vi "test_SomeSessionsRegistered_CallCreateSessions_InitializeCalledWithProperBehavior.vi"(8 "error in":errorcluster) -> (0 "error out":errorcluster, 2 "result":string, 3 "pass":bool)   [LabVIEW 2020, in "MeasurementServerTests.lvlib"]
uses:
  MeasurementServerTests.lvlib
  da6ffb6f-c1c9-4957-84dd-e9228483c454.vi
  ffc64c76-1568-41a3-8328-b9126ac9a28d.vi
  Helpers/Fake Instrument/Fake Instrument.lvclass
  \\tsclient\C/dev/measurementlink-labview/Source/Runtime/MeasurementLink Instrument/IInstrument/IInstrument.lvclass
  Runtime/MeasurementLink Session Management/Session Reservation/Create Sessions Impl.vi
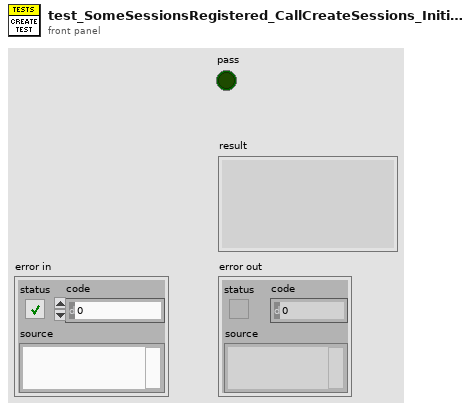
[diagram p1: front panel]
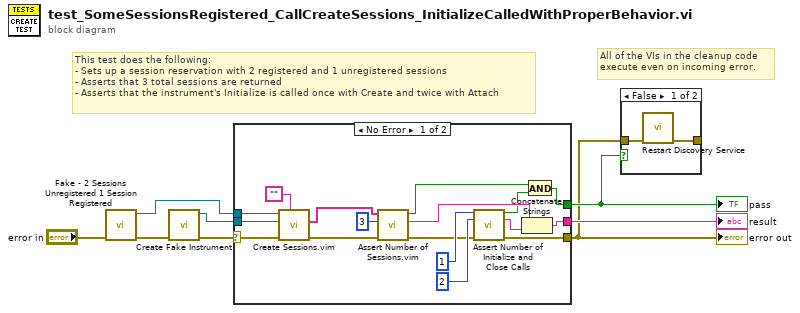
[diagram p0: block diagram]
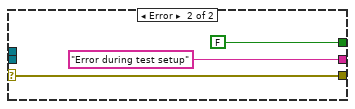
[diagram p2: hidden frame]
diagram:
  # "All of the VIs in the cleanup code\nexecute even on incoming error."
  # "This test does the following:\n- Sets up a session reservation with 2 registered and 1 unregistered sessions\n- Asserts that 3 total sessions are returned\n- Asserts that the instrument's Initialize is called once with Create and twice with Attach"
  n1 = call "Fake - 2 Sessions Unregistered 1 Session Registered.vi"("error in"="error in") -> ("error out"=w2:errorcluster, "session reservation out"=w1:refnum<class "Session Reservation.lvclass">)  [unwired: 9 in]
  n2 = call "Create Fake Instrument.vi"("error in"=w2) -> ("error out"=w5:errorcluster, "fake instrument out"=w4:refnum<class "Fake Instrument.lvclass">)  [unwired: 9 in]
  n3 = case shown="No Error" w5 {
    selector: w5 -> [w23 w26]
    tunnel: [w13 w26] -> w6
    tunnel: [w12 FALSE] -> w7
    tunnel: [w10 "Error during test setup" ("f")] -> w8
    tunnel: w4 -> [w25 _]
    tunnel: w1 -> [w24 _]
    frame No Error {
      n4 = call "Create Sessions.vim"("session type"="", "error in"=w23, "instrument"=w25, "session reservation in"=w24) -> ("error out"=w22:errorcluster, "sessions"=w20:string[])  [unwired: 4 in, 2 out]
      n5 = call "Assert Number of Sessions.vim"("error in"=w22, "expected number of sessions"=3, "sessions"=w20) -> ("error out"=w14:errorcluster, "result"=w19:string, "pass"=w18:bool)  [unwired: 6 in]
      n6 = call "Assert Number of Initialize and Close Calls.vi"("expected initialize-create calls"=u32 1, "expected initialize-attach calls"=u32 2, "error in"=w14) -> ("pass"=w11:bool, "result"=w9:string, "error out"=w13:errorcluster)  [unwired: 10 in]
      n7 = Concatenate Strings(w19, w9) -> (w10:string)
      n8 = And(x=w18, y=w11) -> (x .and. y?=w12:bool)
    }
    frame Error {
    }
  }
  "error out" <- w6
  "pass" <- w7
  "result" <- w8
  n9 = case shown="False" w7 {
    tunnel: w6 -> [w30 _]
    tunnel: [w29 _] -> _
    frame False {
      n10 = call "Restart Discovery Service.vi"("error in"=w30) -> ("error out"=w29:errorcluster)  [unwired: 10 in]
    }
    frame True {
    }
  }
